vi "Normalize.vi"(8 "element 4":dbl, 9 "element 3":dbl, 10 "element 2":dbl, 11 "element 1":dbl) -> (0 "element 4":dbl, 1 "element 3":dbl, 2 "element 2":dbl, 3 "element 1":dbl)   [LabVIEW 2013]
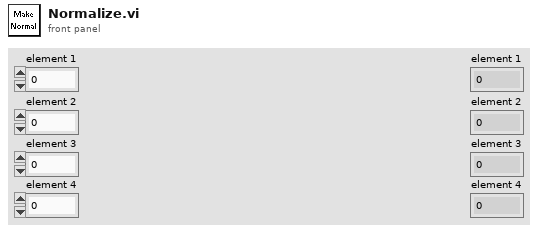
[diagram p1: front panel]
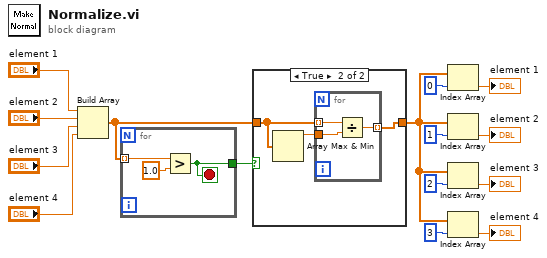
[diagram p0: block diagram]
diagram:
  n1 = Build Array("element 1", "element 2", "element 3", "element 4") -> (w14:dbl[])
  n2 = for {
    tunnel: w14 -> [w18] mode=indexing
    tunnel: [w16] -> w15
    stop <- w16 stop-if-true
    n3 = Greater?(x=w18, y=1.0) -> (0:w16:bool)
  }
  n4 = case shown="True" w15 {
    tunnel: w14 -> [w19 w22]
    tunnel: [w19 w20] -> w9
    frame False {
    }
    frame True {
      n5 = Array Max & Min(array=w22) -> (max value=w21:dbl)  [unwired: 3 out]
      n6 = for {
        tunnel: w22 -> [w25] mode=indexing
        tunnel: w21 -> [w24]
        tunnel: [w23] -> w20 mode=indexing
        n7 = Divide(x=w25, y=w24) -> (x/y=w23:dbl)
      }
    }
  }
  n8 = Index Array(array=w9, index=0) -> (element=→"element 1":dbl)
  n9 = Index Array(array=w9, index=1) -> (element=→"element 2":dbl)
  n10 = Index Array(array=w9, index=2) -> (element=→"element 3":dbl)
  n11 = Index Array(array=w9, index=3) -> (element=→"element 4":dbl)
